vi "G_TMP.vi"() -> ()   [LabVIEW 2018]
panel:
  in  "DMM-dCurrent":dbl
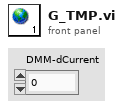
[diagram p1: front panel]
diagram:
